vi "subset_with_SelecteArray.vi"(7 "opt":enum16{"row", "column"}(ring), 10 "Select":i32[](array[numeric]), 11 "X (input Data Array, 2D)":dbl[][](array[numeric])) -> (3 "SubArray":dbl[][](array[numeric]))   [LabVIEW 2014]
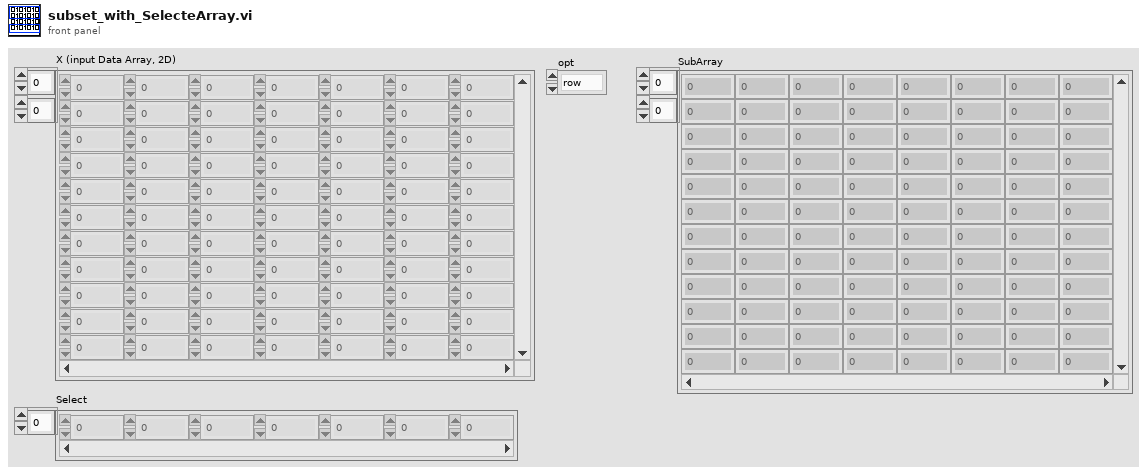
[diagram p1: front panel]
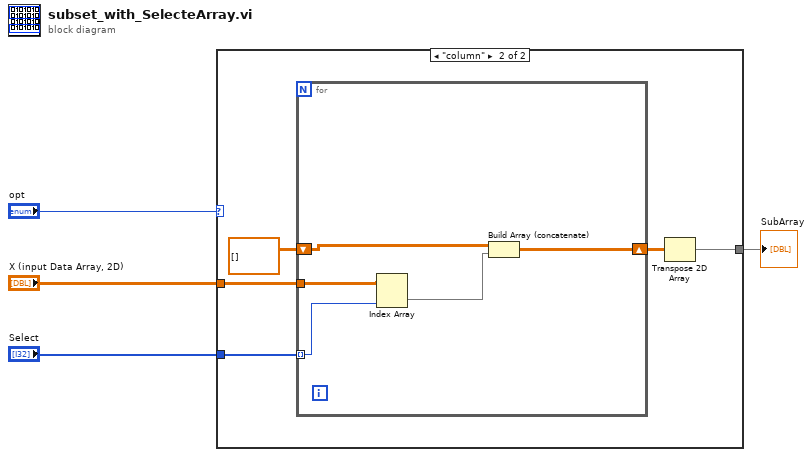
[diagram p0: block diagram]
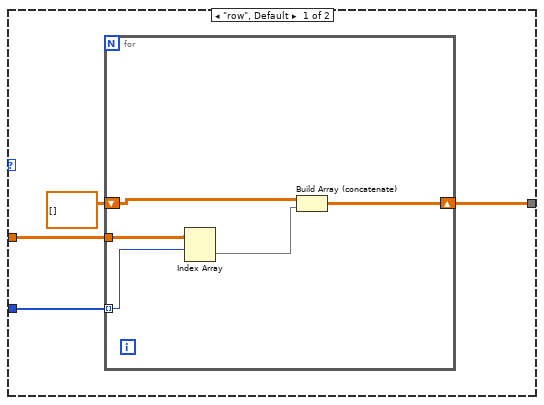
[diagram p2: hidden frame]
diagram:
  n1 = case shown="\"column\"" "opt" {
    tunnel: "X (input Data Array, 2D)" -> [w7 w18]
    tunnel: "Select" -> [w8 w17]
    tunnel: [w5 w14] -> w1
    frame "row", Default {
      n2 = for {
        tunnel: w8 -> [w12] mode=indexing
        tunnel: w7 -> [w13]
        shift-right: [w10] -> w5
        shift-left: dbl[][] [] -> [w9]
        n3 = Index Array(array=w13, index (row)=w12) -> (element=w11:dbl[])  [unwired: 1 in]
        n4 = Build Array (concatenate)(w9, w11) -> (w10:dbl[][])
      }
    }
    frame "column" {
      n5 = for {
        tunnel: w17 -> [w19] mode=indexing
        tunnel: w18 -> [w23]
        shift-right: [w21] -> w15
        shift-left: dbl[][] [] -> [w20]
        n6 = Index Array(array=w23, index (col)=w19) -> (element=w22:dbl[])  [unwired: 1 in]
        n7 = Build Array (concatenate)(w20, w22) -> (w21:dbl[][])
      }
      n8 = Transpose 2D Array(2D array=w15) -> (transposed array=w14:dbl[][])
    }
  }
  "SubArray" <- w1
